vi "Directrion to General Direction.vi"(11 "Direction":T1) -> (3 "General Direction":T1[](array[typedef]))   [LabVIEW 2020]
uses:
  ENUM_Location Direction.ctl
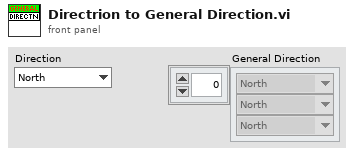
[diagram p1: front panel]
types:
  T1 = typedef "ENUM_Location Direction.ctl" = enum16{"North", "North-East", "East", "South-East", "South", "South-West", "West", "North-West", "Center"}
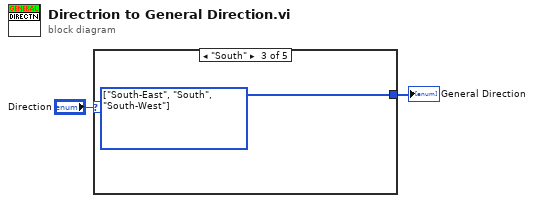
[diagram p0: block diagram]
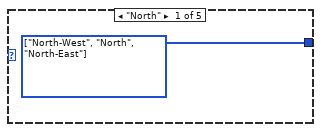
[diagram p2: hidden frame]
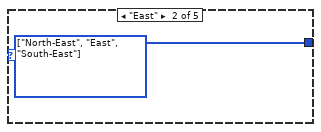
[diagram p3: hidden frame]
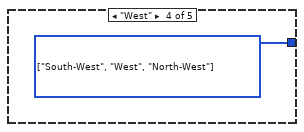
[diagram p4: hidden frame]
diagram:
  n1 = case shown="\"South\"" "Direction" {
    tunnel: [w3 w4 w5 w6 _] -> w2
    frame "North" {
      w3 = T1[] [enum."North-West", enum."North", enum."North-East"] items=["North", "North-East", "East", "South-East", "South", "South-West", "West", "North-West", "Center"] ("List Out")
    }
    frame "East" {
      w4 = T1[] [enum."North-East", enum."East", enum."South-East"] items=["North", "North-East", "East", "South-East", "South", "South-West", "West", "North-West", "Center"] ("List Out")
    }
    frame "South" {
      w5 = T1[] [enum."South-East", enum."South", enum."South-West"] items=["North", "North-East", "East", "South-East", "South", "South-West", "West", "North-West", "Center"] ("List Out")
    }
    frame "West" {
      w6 = T1[] [enum."South-West", enum."West", enum."North-West"] items=["North", "North-East", "East", "South-East", "South", "South-West", "West", "North-West", "Center"] ("List Out")
    }
    frame Default {
    }
  }
  "General Direction" <- w2
